vi "Convert PNG color.vi"(7 "New Color":u32(colorbox)=14450432, 8 "error in":errorcluster, 10 "new file":path, 11 "orig file":path) -> (0 "error out":errorcluster, 2 "new file out":path, 3 "orig file out":path)   [LabVIEW 2021, in "TSC Material Theme.lvlib" / "Material-Scheme.lvclass"]
doc: "Change the colors of the png file using .net functions\n\n<b>Note</b>: Assumes a single color PNG file - replace old primary with new primary\n\n<b>Code Developed By:</b>\nTechnology Service Corporation\nwww.tsc.com/atcs\n\nDeveloper:\nDaniel Coons"
uses:
  Material-Scheme.lvclass
  System.Drawing
  Material-Scheme.lvclass/Material-Scheme.ctl
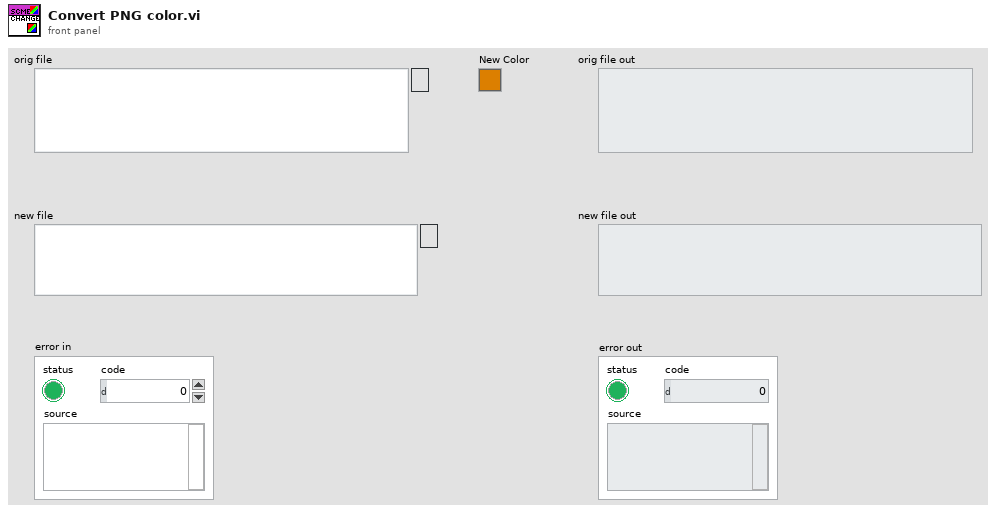
[diagram p1: front panel]
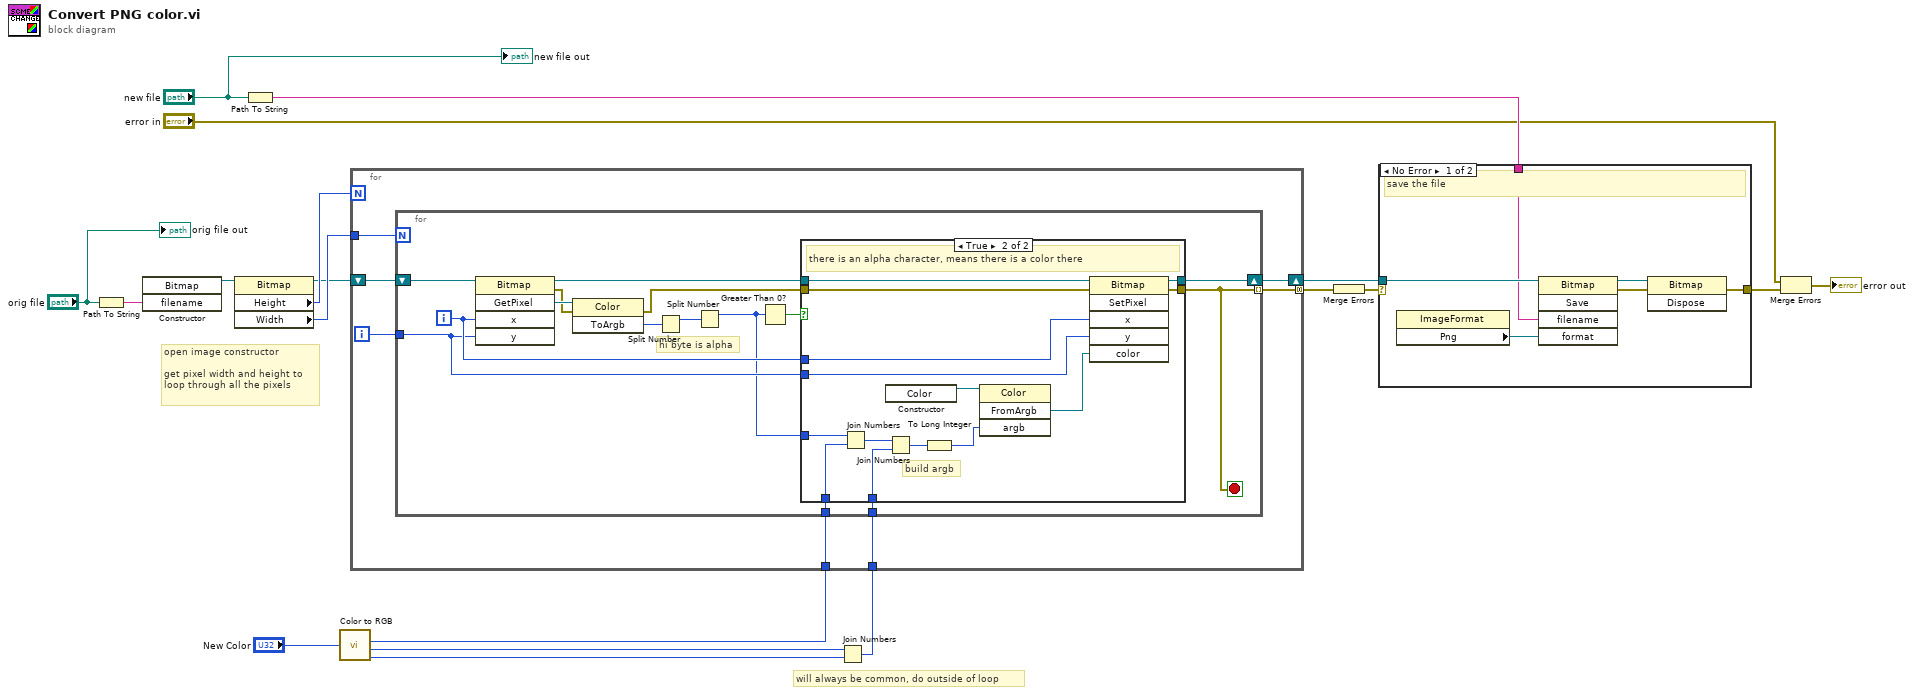
[diagram p0: block diagram]
diagram:
  # "will always be common, do outside of loop"
  # "open image constructor\n\nget pixel width and height to \nloop through all the pixels"
  n1 = Path To String(path="orig file") -> (string=w19:string)
  n2 = constructor class="Bitmap"("filename"=w19) -> (reference out=w18:refnum<k24>)  [unwired: 3 in, 3 out]
  n3 = property class="Bitmap"(reference=w18) -> (reference out=w15:refnum<k24>, "Height"=w17:i32, "Width"=w16:i32)  [unwired: 1 in, 1 out]
  n4 = Path To String(path="new file") -> (string=w13:string)
  n5 = call <vilib>:"Color to RGB.vi"("Color"="New Color") -> ("R"=w10:u8, "G"=w8:u8, "B"=w7:u8)  [unwired: 1 out]
  n6 = Join Numbers(hi=w8, lo=w7) -> ((hi.lo)=w9:u16)
  n7 = for {
    N: w17 -> [_]
    tunnel: w16 -> [w26]
    shift-right: [w23] -> w14
    shift-left: w15 -> [w24]
    tunnel: w10 -> [w22]
    tunnel: w9 -> [w21]
    tunnel: [w20] -> w6 mode=concatenating
    i -> [w25]
    n8 = for {
      N: w26 -> [_]
      tunnel: w25 -> [w37]
      shift-right: [w36] -> w23
      shift-left: w24 -> [w40]
      tunnel: w22 -> [w29]
      tunnel: w21 -> [w28]
      tunnel: [w27] -> w20 mode=indexing
      i -> [w38]
      stop <- w27 stop-if-true
      # "hi byte is alpha"
      n9 = invoke class="Bitmap" method="GetPixel"(reference=w40, "x"=w38, "y"=w37) -> (reference out=w39:refnum<k24>, error out=w31:errorcluster, "GetPixel"=w41:refnum<k24>)  [unwired: 2 in, 2 out]
      n10 = invoke class="Color" method="ToArgb"(reference=w41, error in=w31) -> (error out=w30:errorcluster, "ToArgb"=w32:i32)  [unwired: 1 in, 1 out]
      n11 = Split Number(x=w32) -> (hi(x)=w35:u16)  [unwired: 1 out]
      n12 = Split Number(x=w35) -> (hi(x)=w33:u8)  [unwired: 1 out]
      n13 = Greater Than 0?(x=w33) -> (x > 0?=w34:bool)
      n14 = case shown="True" w34 {
        tunnel: w39 -> [w43 w57]
        tunnel: w38 -> [_ w56]
        tunnel: w37 -> [_ w55]
        tunnel: [w43 w54] -> w36
        tunnel: w33 -> [_ w51]
        tunnel: w30 -> [w42 w48]
        tunnel: w29 -> [_ w47]
        tunnel: w28 -> [_ w45]
        tunnel: [w42 w44] -> w27
        frame False {
          # "no alpha, no change"
        }
        frame True {
          # "build argb"
          # "there is an alpha character, means there is a color there"
          n15 = Join Numbers(hi=w51, lo=w47) -> ((hi.lo)=w50:u16)
          n16 = constructor class="Color"() -> (reference out=w53:refnum<k24>)  [unwired: 3 in, 2 out]
          n17 = Join Numbers(hi=w50, lo=w45) -> ((hi.lo)=w49:u32)
          n18 = To Long Integer(number=w49) -> (32bit integer=w46:i32)
          n19 = invoke class="Color" method="FromArgb"(reference=w53, "argb"=w46) -> ("FromArgb"=w52:refnum<k24>)  [unwired: 2 in, 3 out]
          n20 = invoke class="Bitmap" method="SetPixel"(reference=w57, error in=w48, "x"=w56, "y"=w55, "color"=w52) -> (reference out=w54:refnum<k24>, error out=w44:errorcluster)  [unwired: 1 in, 4 out]
        }
      }
    }
  }
  n21 = Merge Errors(w6) -> (w5:errorcluster)
  n22 = case shown="No Error" w5 {
    selector: w5 -> [_ w64]
    tunnel: w14 -> [w63 _]
    tunnel: w13 -> [w62 _]
    tunnel: [w61 w64] -> w12
    frame No Error {
      # "save the file"
      n23 = property class="ImageFormat"() -> ("Png"=w59:refnum<k24>)  [unwired: 2 in, 2 out]
      n24 = invoke class="Bitmap" method="Save"(reference=w63, "filename"=w62, "format"=w59) -> (reference out=w58:refnum<k24>, error out=w60:errorcluster)  [unwired: 2 in, 3 out]
      n25 = invoke class="Bitmap" method="Dispose"(reference=w58, error in=w60) -> (error out=w61:errorcluster)  [unwired: 1 in, 2 out]
    }
    frame Error {
    }
  }
  n26 = Merge Errors("error in", w12) -> (→"error out":errorcluster)
  "orig file out" <- "orig file"
  "new file out" <- "new file"
